vi "Group_Set_MetaData.vi"(8 "error in (no error)":errorcluster, 10 "Meta Data":T1[](array[typedef]), 11 "Group in":refnum<class "Group.lvclass">) -> (0 "error out":errorcluster, 3 "Group out":refnum<class "Group.lvclass">)   [LabVIEW 2023, in "Group.lvclass"]
doc: "Sets the meta data on the group level as a property name and value key pairing."
uses:
  Group.lvclass
  Meta Data.ctl
  Group.lvclass/Group.ctl
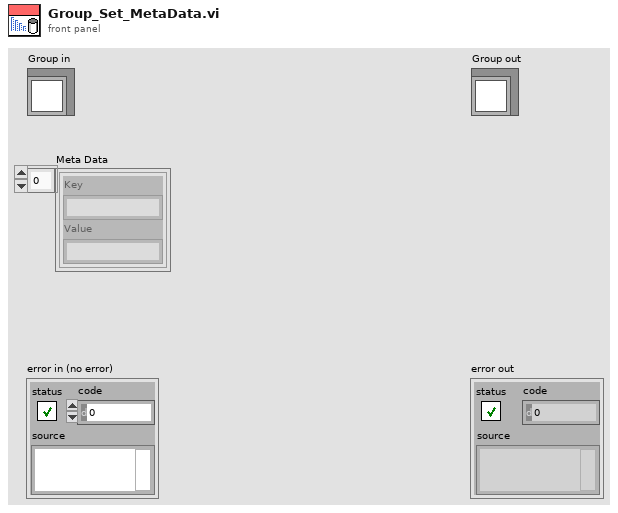
[diagram p1: front panel]
types:
  T1 = typedef "Meta Data.ctl" = cluster{"Key":string, "Value":string}
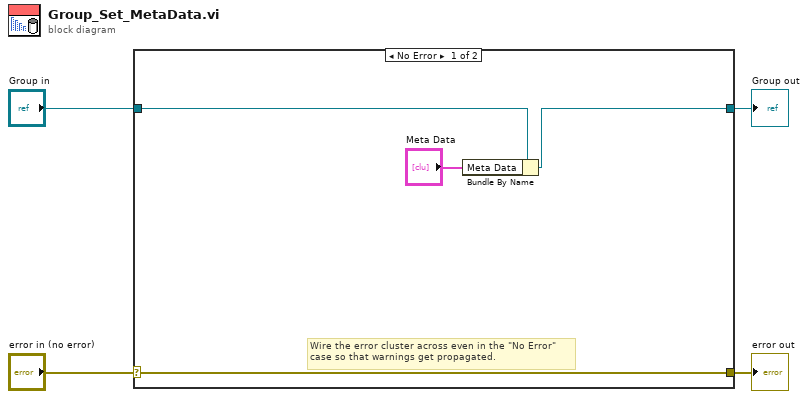
[diagram p0: block diagram]
diagram:
  n1 = case shown="No Error" "error in (no error)" {
    selector: "error in (no error)" -> [w8 w10]
    tunnel: [w8 w10] -> w3
    tunnel: [w6 w9] -> w1
    tunnel: "Group in" -> [w7 w9]
    frame No Error {
      # "Wire the error cluster across even in the \"No Error\"\ncase so that warnings get propagated."
      n2 = Bundle By Name(cluster=w7, "Meta Data"="Meta Data") -> (w6:refnum<class "Group.lvclass">)
    }
    frame Error {
    }
  }
  "error out" <- w3
  "Group out" <- w1
